vi "Generate Population.vi"(8 "error in (no error)":errorcluster, 9 "seed":i32=-1, 10 "OSSP_Problem.lvclass":refnum<class "OSSP_Problem.lvclass">, 11 "GA in":refnum<class "GA.lvclass">) -> (0 "error out":errorcluster, 3 "GA out":refnum<class "GA.lvclass">)   [LabVIEW 2013, in "GA.lvclass"]
uses:
  GA.lvclass
  OSSP_Problem.lvclass
  GA.lvclass/GA.ctl
  Controls/Solution_GA.ctl
  OSSP_Problem.lvclass/OSSP_Problem.ctl
  Helper VIs/IRH Heuristic VIs/Initial Construction Heuristic.ctl
  GA/Controls/Scheduler Type.ctl
  Scheduler_Class/Prins FIFO Scheduler Methods and Controls/Prins FIFO Scheduler.vi
  Scheduler_Class/Prins FIFO Scheduler Methods and Controls/Methods/Calculate Final Completion Times of Jobs.vi
  Scheduler_Class/Prins FIFO Scheduler Methods and Controls/Methods/Reorder Schedule(Prins FIFO) based on Start Times.vi
  OSSP_Problem_Class/Getters/Read Number of Jobs.vi
  OSSP_Problem_Class/Getters/Read Number of Machines.vi
  Scheduler_Class/NonDelay Scheduler/Non Delay Scheduler Engine.vi
  OSSP_Problem_Class/Getters/Read Due Dates.vi
  Scheduler_Class/Operation to Machine Job Tuple.vi
  <vilib>/dlg_ctls.llb/Space Constant.vi
  GA/SubVIS/Calcualte General Tardiness.vi
  Helper VIs/IRH Heuristic VIs/LPTSequenceBulilder.vi
  Helper VIs/IRH Heuristic VIs/SPTSequenceBulilder.vi
  Helper VIs/IRH Heuristic VIs/EDDSequenceBulilder.vi
  Scheduler_Class/Prins FIFO Scheduler Methods and Controls/Methods/UpdateMachineGaps.vi
  Scheduler_Class/Prins FIFO Scheduler Methods and Controls/Methods/UpdateJobGaps.vi
  Scheduler_Class/Prins FIFO Scheduler Methods and Controls/Methods/Find Intersecting Gaps.vi
  <vilib>/Analysis/1siggen.llb/Riffle Array (I32).vi
  Scheduler_Class/Prins FIFO Scheduler Methods and Controls/Methods/Transform to Plain Job and Machine Gaps Array.vi
  <vilib>/Analysis/NI_AALBase.lvlib
  Scheduler.lvclass
panel:
  out "Total Tardiness EDD":u16
  out "Total Tardiness SPT":u16
  out "Total Tardiness LPT":u16
  out "Schedule Out":i32[](array[numeric])
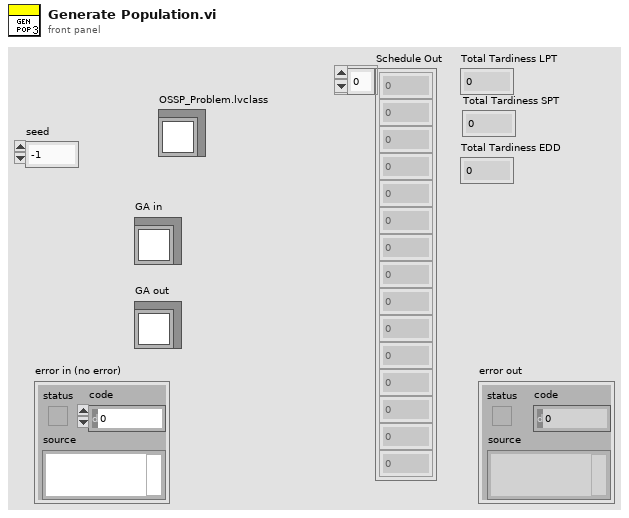
[diagram p1: front panel]
types:
  T1 = typedef "Solution_GA.ctl" = cluster{"Schedule":u16[], "Fitness":u16, "Fitness Valid?":bool}
  T2 = enum16{"Semi Active Scheduler", "Non Delay Scheduler"}
  T3 = typedef "Initial Construction Heuristic.ctl" = enum16{"LPT", "SPT", "EDD"}
  T4 = typedef "Objective.ctl" = enum16{"Makespan", "Total Tardiness"}
  T5 = typedef "GA.lvclass/Initial Population Generation.ctl" = enum16{"Random", "Heuristic Solution"}
  T6 = typedef "Scheduler Type.ctl" = enum16{"Non Delay Scheduler", "GT Active Scheduler", "My Faulty Scheduler", "Prins FIFO Scheduler", "SemiActive Scheduler"}
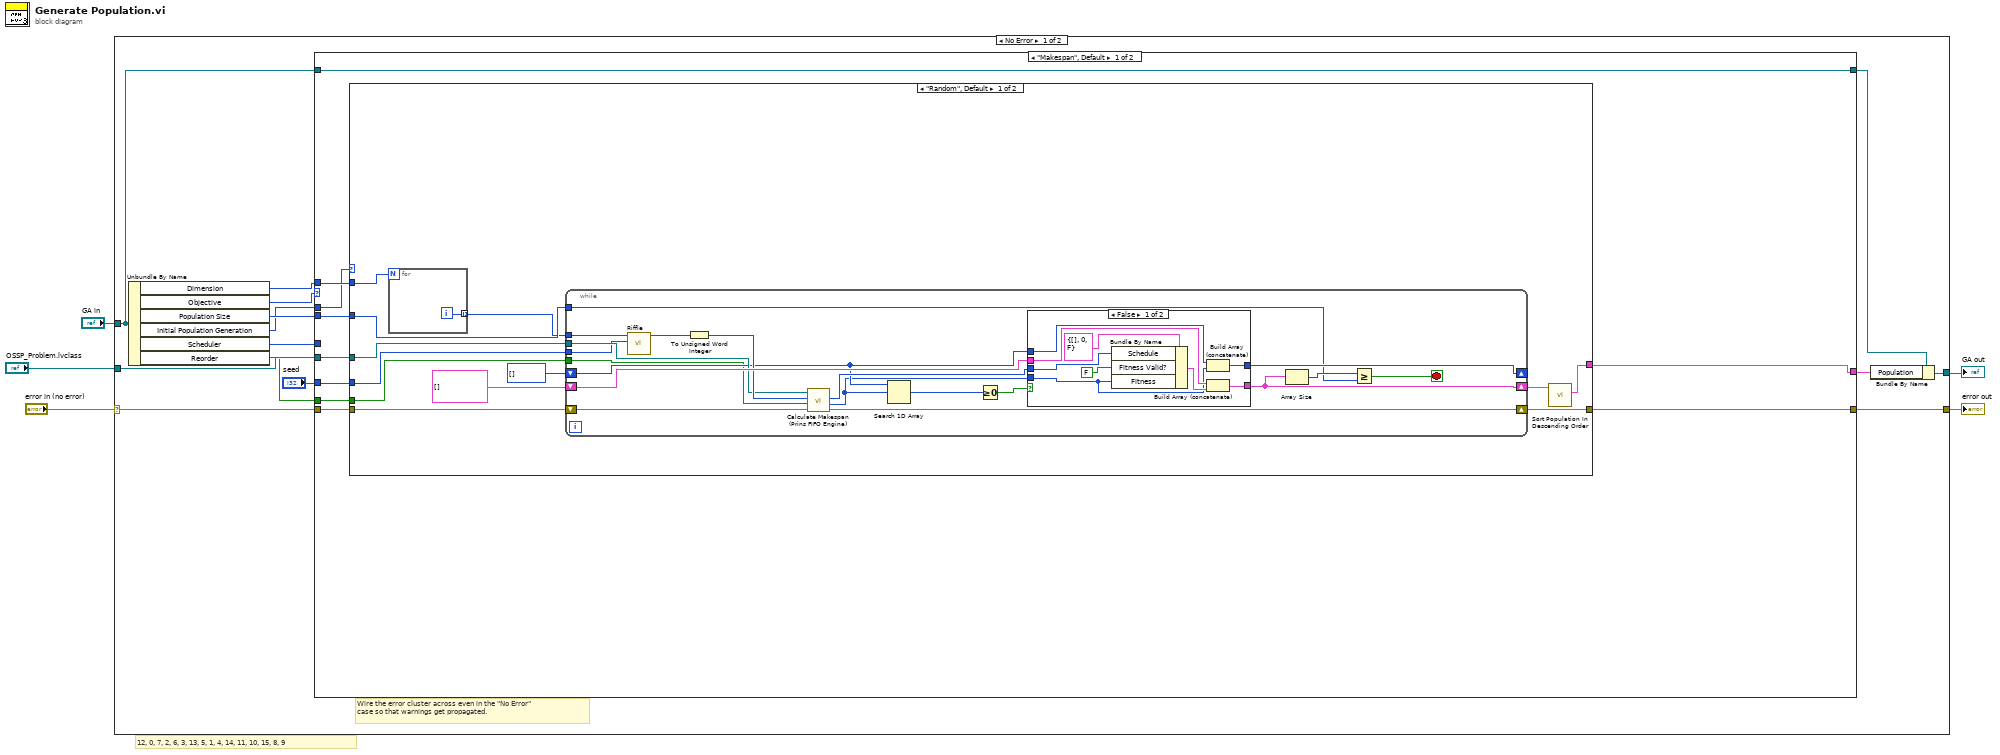
[diagram p0: block diagram]
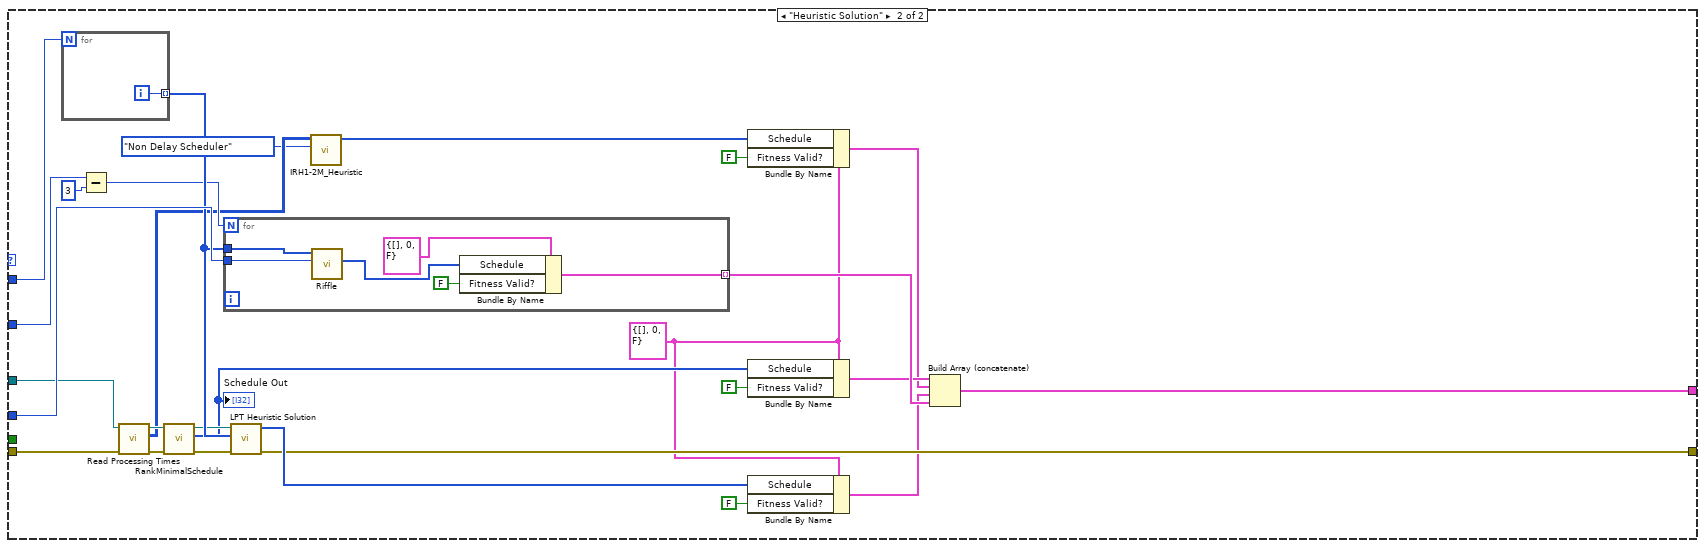
[diagram p3: hidden frame]
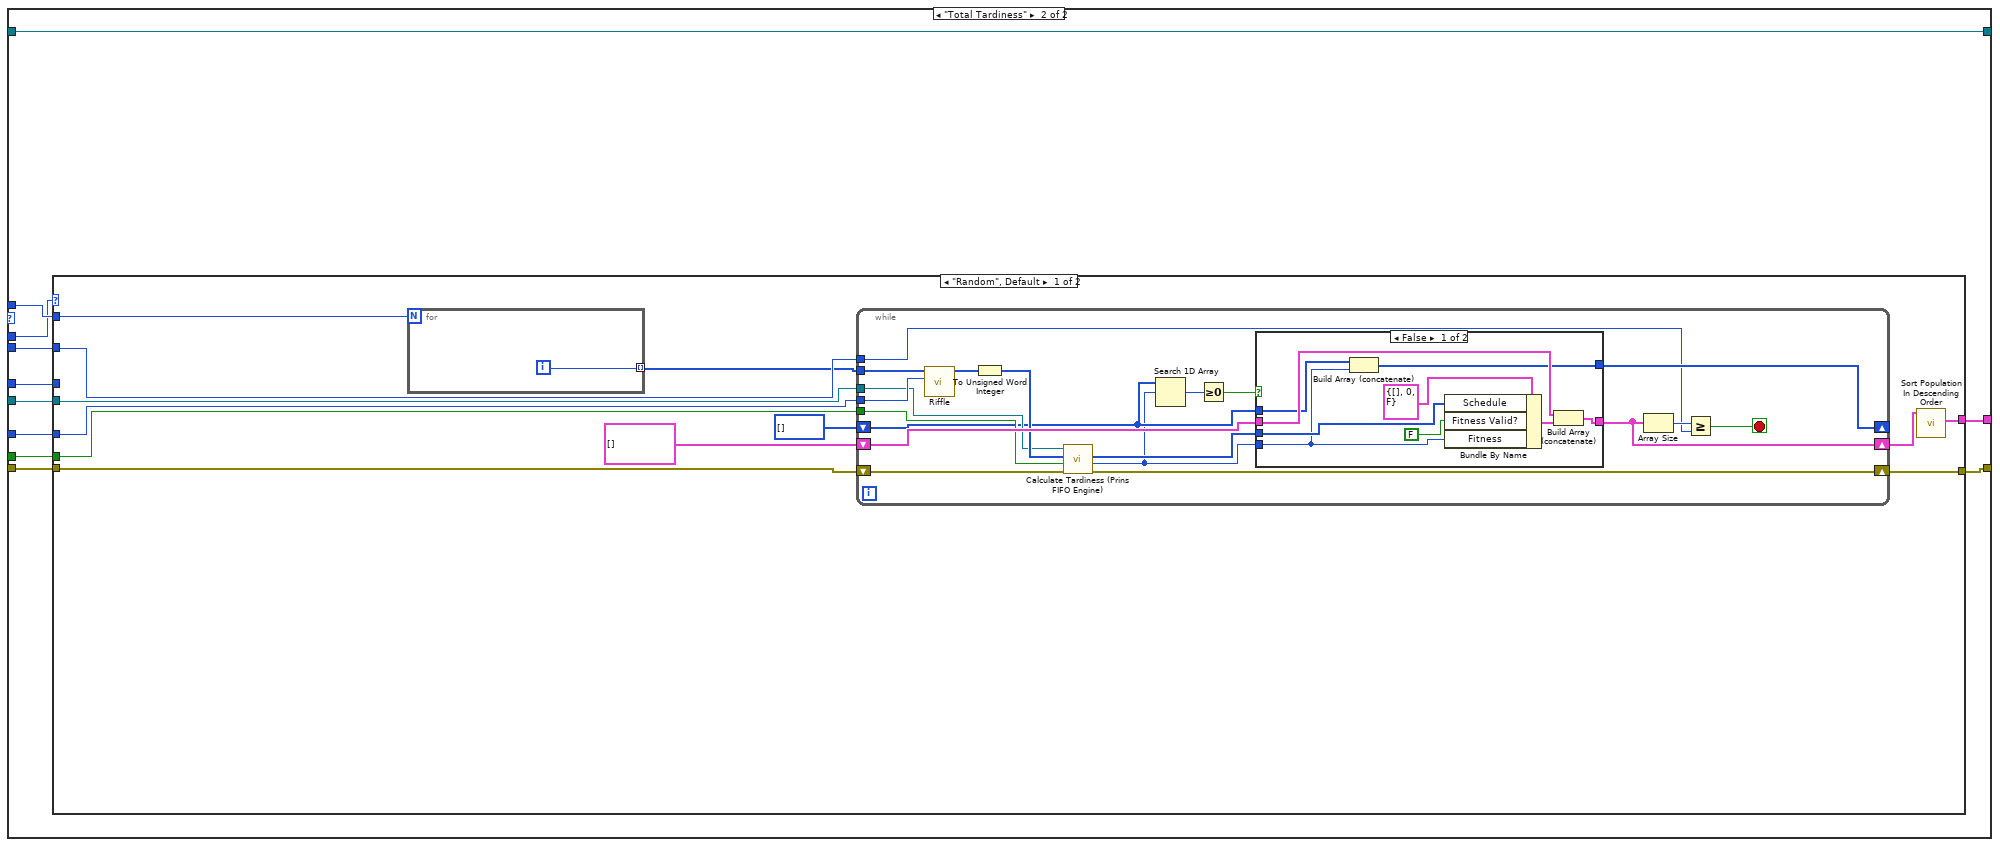
[diagram p4: hidden frame]
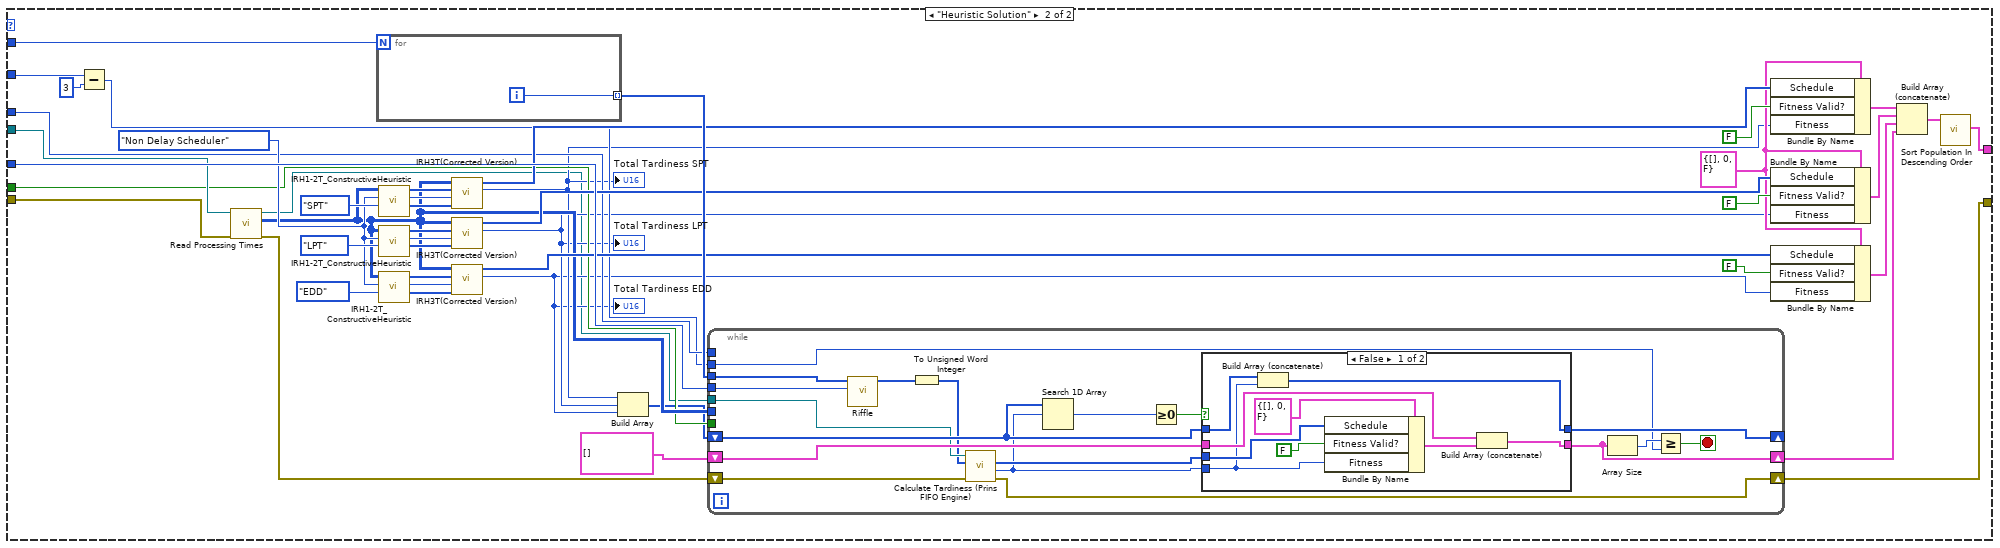
[diagram p6: hidden frame]
diagram:
  # "12, 0, 7, 2, 6, 3, 13, 5, 1, 4, 14, 11, 10, 15, 8, 9"
  n1 = case shown="No Error" "error in (no error)" {
    selector: "error in (no error)" -> [w12 w237]
    tunnel: [w14 w237] -> w4
    tunnel: [w18 w236] -> w2
    tunnel: "GA in" -> [w10 w236]
    tunnel: "OSSP_Problem.lvclass" -> [w11 _]
    frame No Error {
      # "Wire the error cluster across even in the \"No Error\"\ncase so that warnings get propagated."
      n2 = Unbundle By Name(w10) -> ("Dimension"=w19:i32, "Objective"=w15:T4, "Population Size"=w13:u32, "Initial Population Generation"=w8:T5, "Scheduler"=w7:T6, "Reorder"=w6:bool)
      n3 = case shown="\"Makespan\", Default" w15 {
        tunnel: w19 -> [w29 w117]
        tunnel: "seed" -> [w28 w116]
        tunnel: [w27 w114] -> w16
        tunnel: w11 -> [w24 w112]
        tunnel: w12 -> [w23 w115]
        tunnel: [w26 w111] -> w14
        tunnel: w13 -> [w25 w113]
        tunnel: w10 -> [w22 w110]
        tunnel: [w22 w110] -> w9
        tunnel: w8 -> [w21 w109]
        tunnel: w7 -> [_ w108]
        tunnel: w6 -> [w20 w107]
        frame "Makespan", Default {
          n4 = case shown="\"Random\", Default" w21 {
            tunnel: w29 -> [w33 w99]
            tunnel: w28 -> [w32 w98]
            tunnel: [w30 w95] -> w27
            tunnel: [w40 w92] -> w26
            tunnel: w25 -> [w38 w86]
            tunnel: w24 -> [w39 w83]
            tunnel: w23 -> [w41 w82]
            tunnel: w20 -> [w31 _]
            frame "Random", Default {
              n5 = for {
                N: w33 -> [_]
                tunnel: [w72] -> w37 mode=indexing
                i -> [w72]
              }
              n6 = while {
                tunnel: w37 -> [w60]
                tunnel: w38 -> [w50]
                shift-right: [w51] -> w34
                shift-left: T1[] [] -> [w53]
                shift-right: [w52] -> _
                shift-left: u16[] [] ("appended array") -> [w45]
                shift-right: [w48] -> w40
                shift-left: w41 -> [w49]
                tunnel: w39 -> [w46]
                tunnel: w32 -> [w43]
                tunnel: w31 -> [w42]
                stop <- w56 stop-if-true
                n7 = call-poly <vilib>:"Riffle.vi"("seed"=w43, "X"=w60) -> ("Riffled {X}"=w58:i32[])  [unwired: 7 in, 2 out]
                n8 = To Unsigned Word Integer(number=w58) -> (unsigned 16bit integer=w47:u16[])
                n9 = call "Calculate Makespan (Prins FIFO Engine).vi"("error in (no error)"=w49, "Reorder?"=w42, "Schedule In"=w47, "OSSP_Problem in"=w46) -> ("error out"=w48:errorcluster, "Makespan"=w44:i32, "Schedule Out"=w59:u16[])  [unwired: 4 in, 1 out]
                n10 = Search 1D Array(1D array=w45, element=w44) -> (index of element=w55:i32)  [unwired: 1 in]
                n11 = Greater Or Equal To 0?(x=w55) -> (x >= 0?=w54:bool)
                n12 = case shown="False" w54 {
                  tunnel: w59 -> [w67 _]
                  tunnel: w53 -> [w66 w71]
                  tunnel: [w64 w71] -> w51
                  tunnel: w45 -> [w63 w70]
                  tunnel: [w62 w70] -> w52
                  tunnel: w44 -> [w61 _]
                  frame False {
                    n13 = Bundle By Name(cluster=T1 {"Schedule"=[], "Fitness"=0, "Fitness Valid?"=FALSE} ("Solution"), "Schedule"=w67, "Fitness Valid?"=FALSE, "Fitness"=w61) -> (w65:T1)
                    n14 = Build Array (concatenate)(w63, w61) -> (w62:i32[])
                    n15 = Build Array (concatenate)(w66, w65) -> (w64:T1[])
                  }
                  frame True {
                  }
                }
                n16 = Array Size(array=w51) -> (size(s)=w57:i32)
                n17 = Greater Or Equal?(x=w57, y=w50) -> (x >= y?=w56:bool)
              }
              n18 = call "Sort Population In Descending Order.vi"("Population"=w34) -> ("Population In Descending Order"=w30:T1[])  [unwired: 9 in, 1 out]
            }
            frame "Heuristic Solution" {
              w77 = T1 {"Schedule"=[], "Fitness"=0, "Fitness Valid?"=FALSE} ("Solution")
              n19 = for {
                N: w99 -> [_]
                tunnel: [w100] -> w97 mode=indexing
                i -> [w100]
              }
              n20 = Subtract(x=w86, y=u8 3) -> (x-y=w84:u32)
              n21 = call "Read Processing Times.vi"("error in (no error)"=w82, "OSSP_Problem in"=w83) -> ("error out"=w81:errorcluster, "Processing Times"=w79:u16[][], "OSSP_Problem out"=w80:refnum<class "OSSP_Problem.lvclass">)  [unwired: 7 in]
              n22 = call "RankMinimalSchedule.vi"("error in (no error)"=w81, "OSSP_Problem in"=w80) -> ("error out"=w91:errorcluster, "Schedule Out"=w89:i32[], "OSSP_Problem out"=w90:refnum<class "OSSP_Problem.lvclass">)  [unwired: 7 in]
              "Schedule Out" <- w89
              n23 = for {
                N: w84 -> [_]
                tunnel: w97 -> [w106]
                tunnel: w98 -> [w105]
                tunnel: [w103] -> w96 mode=indexing
                n24 = call-poly <vilib>:"Riffle.vi"("seed"=w105, "X"=w106) -> ("Riffled Index"=w104:i32[])  [unwired: 7 in, 2 out]
                n25 = Bundle By Name(cluster=T1 {"Schedule"=[], "Fitness"=0, "Fitness Valid?"=FALSE} ("Solution"), "Schedule"=w104, "Fitness Valid?"=FALSE) -> (w103:T1)
              }
              n26 = call "LPT Heuristic Solution.vi"("error in (no error)"=w91, "Array"=w97, "OSSP_Problem in"=w90) -> ("error out"=w92:errorcluster, "LPT List Heuristic Solution"=w93:u16[])  [unwired: 7 in]
              n27 = call "IRH1-2M_Heuristic.vi"("Scheduler"=T2."Non Delay Scheduler", "Proocessing Times"=w79) -> ("IRH1 Schedule"=w73:u16[])  [unwired: 9 in]
              n28 = Bundle By Name(cluster=w77, "Schedule"=w73, "Fitness Valid?"=FALSE) -> (w75:T1)
              n29 = Bundle By Name(cluster=w77, "Schedule"=w89, "Fitness Valid?"=FALSE) -> (w87:T1)
              n30 = Bundle By Name(cluster=w77, "Schedule"=w93, "Fitness Valid?"=FALSE) -> (w74:T1)
              n31 = Build Array (concatenate)(w87, w75, w74, w96) -> (w95:T1[])
            }
          }
        }
        frame "Total Tardiness" {
          n32 = case shown="\"Random\", Default" w109 {
            tunnel: w117 -> [w129 w205]
            tunnel: w116 -> [w127 w204]
            tunnel: w115 -> [w124 w174]
            tunnel: [w122 w164] -> w114
            tunnel: w113 -> [w126 w203]
            tunnel: w112 -> [w125 w202]
            tunnel: [w123 w161] -> w111
            tunnel: w108 -> [_ w176]
            tunnel: w107 -> [w128 w173]
            frame "Random", Default {
              n33 = for {
                N: w129 -> [_]
                tunnel: [w160] -> w121 mode=indexing
                i -> [w160]
              }
              n34 = while {
                tunnel: w121 -> [w148]
                tunnel: w127 -> [w147]
                tunnel: w128 -> [w132]
                tunnel: w126 -> [w137]
                shift-right: [w138] -> w118
                shift-left: T1[] [] -> [w140]
                shift-right: [w139] -> _
                shift-left: u16[] [] ("appended array") -> [w131]
                shift-right: [w135] -> w123
                shift-left: w124 -> [w136]
                tunnel: w125 -> [w133]
                stop <- w143 stop-if-true
                n35 = call-poly <vilib>:"Riffle.vi"("seed"=w147, "X"=w148) -> ("Riffled {X}"=w145:i32[])  [unwired: 7 in, 2 out]
                n36 = To Unsigned Word Integer(number=w145) -> (unsigned 16bit integer=w134:u16[])
                n37 = call "Calculate Tardiness (Prins FIFO Engine).vi"("error in (no error)"=w136, "Reorder?"=w132, "Schedule In"=w134, "OSSP_Problem in"=w133) -> ("error out"=w135:errorcluster, "Tardiness(Prins FIFO Engine)"=w130:u16, "Schedule Out"=w146:u16[])  [unwired: 3 in, 2 out]
                n38 = Search 1D Array(1D array=w131, element=w130) -> (index of element=w142:i32)  [unwired: 1 in]
                n39 = Greater Or Equal To 0?(x=w142) -> (x >= 0?=w141:bool)
                n40 = case shown="False" w141 {
                  tunnel: w146 -> [w155 _]
                  tunnel: w140 -> [w154 w159]
                  tunnel: [w152 w159] -> w138
                  tunnel: w131 -> [w151 w158]
                  tunnel: [w150 w158] -> w139
                  tunnel: w130 -> [w149 _]
                  frame False {
                    n41 = Build Array (concatenate)(w151, w149) -> (w150:u16[])
                    n42 = Bundle By Name(cluster=T1 {"Schedule"=[], "Fitness"=0, "Fitness Valid?"=FALSE} ("Solution"), "Schedule"=w155, "Fitness Valid?"=FALSE, "Fitness"=w149) -> (w153:T1)
                    n43 = Build Array (concatenate)(w154, w153) -> (w152:T1[])
                  }
                  frame True {
                  }
                }
                n44 = Array Size(array=w138) -> (size(s)=w144:i32)
                n45 = Greater Or Equal?(x=w144, y=w137) -> (x >= y?=w143:bool)
              }
              n46 = call "Sort Population In Descending Order.vi"("Population"=w118) -> ("Population In Descending Order"=w122:T1[])  [unwired: 9 in, 1 out]
            }
            frame "Heuristic Solution" {
              w178 = Scheduler_Type."Non Delay Scheduler" ("Scheduler")
              w177 = T1 {"Schedule"=[], "Fitness"=0, "Fitness Valid?"=FALSE} ("Solution")
              n47 = Subtract(x=w203, y=u8 3) -> (x-y=w172:u32)
              n48 = call "Read Processing Times.vi"("error in (no error)"=w174, "OSSP_Problem in"=w202) -> ("error out"=w162:errorcluster, "Processing Times"=w175:u16[][], "OSSP_Problem out"=w163:refnum<class "OSSP_Problem.lvclass">)  [unwired: 7 in]
              n49 = for {
                N: w205 -> [_]
                tunnel: [w235] -> w201 mode=indexing
                i -> [w235]
              }
              n50 = call "IRH1-2T_ConstructiveHeuristic.vi"("Initial Construction Heursitic"=Initial_Construction_Heuristic."SPT", "Scheduler"=w178, "Proocessing Times MxJ"=w175) -> ("Due Dates"=w191:u16[], "Total Tardiness"=w192:u16, "IRH2T Schedule Out"=w193:u16[])  [unwired: 6 in]
              n51 = call "IRH1-2T_ConstructiveHeuristic.vi"("Initial Construction Heursitic"=Initial_Construction_Heuristic."LPT", "Scheduler"=w178, "Proocessing Times MxJ"=w175) -> ("Due Dates"=w196:u16[], "Total Tardiness"=w197:u16, "IRH2T Schedule Out"=w198:u16[])  [unwired: 6 in]
              n52 = call "IRH1-2T_ConstructiveHeuristic.vi"("Initial Construction Heursitic"=Initial_Construction_Heuristic."EDD", "Scheduler"=w178, "Proocessing Times MxJ"=w175) -> ("Due Dates"=w187:u16[], "Total Tardiness"=w188:u16, "IRH2T Schedule Out"=w189:u16[])  [unwired: 6 in]
              n53 = call "IRH3T(Corrected Version).vi"("Due Dates"=w191, "Initial Tardiness"=w192, "Schedule 2B Improved"=w193, "Proocessing Times  (Machines x Jobs)"=w175) -> ("Total Tardiness"=w169:u16, "IRH3T (Reordered) Schedule Out"=w183:u16[])  [unwired: 5 in, 1 out]
              "Total Tardiness SPT" <- w169
              n54 = call "IRH3T(Corrected Version).vi"("Due Dates"=w196, "Initial Tardiness"=w197, "Schedule 2B Improved"=w198, "Proocessing Times  (Machines x Jobs)"=w175) -> ("Total Tardiness"=w168:u16, "IRH3T (Reordered) Schedule Out"=w184:u16[])  [unwired: 5 in, 1 out]
              "Total Tardiness LPT" <- w168
              n55 = call "IRH3T(Corrected Version).vi"("Due Dates"=w187, "Initial Tardiness"=w188, "Schedule 2B Improved"=w189, "Proocessing Times  (Machines x Jobs)"=w175) -> ("Total Tardiness"=w167:u16, "IRH3T (Reordered) Schedule Out"=w182:u16[])  [unwired: 5 in, 1 out]
              "Total Tardiness EDD" <- w167
              n56 = Build Array(w169, w168, w167) -> (w166:u16[])
              n57 = while {
                tunnel: w201 -> [w223]
                tunnel: w204 -> [w222]
                tunnel: w176 -> [_]
                tunnel: w175 -> [_]
                tunnel: w163 -> [w210]
                tunnel: w173 -> [_]
                tunnel: w172 -> [w211]
                shift-right: [w212] -> w170
                shift-left: T1[] [] -> [w215]
                shift-right: [w213] -> _
                shift-left: w166 -> [w214]
                shift-right: [w208] -> w161
                shift-left: w162 -> [w209]
                stop <- w218 stop-if-true
                n58 = call-poly <vilib>:"Riffle.vi"("seed"=w222, "X"=w223) -> ("Riffled {X}"=w220:i32[])  [unwired: 7 in, 2 out]
                n59 = To Unsigned Word Integer(number=w220) -> (unsigned 16bit integer=w207:u16[])
                n60 = call "Calculate Tardiness (Prins FIFO Engine).vi"("error in (no error)"=w209, "Schedule In"=w207, "OSSP_Problem in"=w210) -> ("error out"=w208:errorcluster, "Tardiness(Prins FIFO Engine)"=w206:u16, "Schedule Out"=w221:u16[])  [unwired: 4 in, 2 out]
                n61 = Search 1D Array(1D array=w214, element=w206) -> (index of element=w217:i32)  [unwired: 1 in]
                n62 = Greater Or Equal To 0?(x=w217) -> (x >= 0?=w216:bool)
                n63 = case shown="False" w216 {
                  tunnel: w221 -> [w230 _]
                  tunnel: w215 -> [w229 w234]
                  tunnel: [w227 w234] -> w212
                  tunnel: w214 -> [w226 w233]
                  tunnel: [w225 w233] -> w213
                  tunnel: w206 -> [w224 _]
                  frame False {
                    n64 = Build Array (concatenate)(w226, w224) -> (w225:u16[])
                    n65 = Bundle By Name(cluster=T1 {"Schedule"=[], "Fitness"=0, "Fitness Valid?"=FALSE} ("Solution"), "Schedule"=w230, "Fitness Valid?"=FALSE, "Fitness"=w224) -> (w228:T1)
                    n66 = Build Array (concatenate)(w229, w228) -> (w227:T1[])
                  }
                  frame True {
                  }
                }
                n67 = Array Size(array=w212) -> (size(s)=w219:i32)
                n68 = Greater Or Equal?(x=w219, y=w211) -> (x >= y?=w218:bool)
              }
              n69 = Bundle By Name(cluster=w177, "Schedule"=w183, "Fitness Valid?"=FALSE, "Fitness"=w169) -> (w180:T1)
              n70 = Bundle By Name(cluster=w177, "Schedule"=w184, "Fitness Valid?"=FALSE, "Fitness"=w168) -> (w179:T1)
              n71 = Bundle By Name(cluster=w177, "Schedule"=w182, "Fitness Valid?"=FALSE, "Fitness"=w167) -> (w181:T1)
              n72 = Build Array (concatenate)(w180, w179, w181, w170) -> (w165:T1[])
              n73 = call "Sort Population In Descending Order.vi"("Population"=w165) -> ("Population In Descending Order"=w164:T1[])  [unwired: 9 in, 1 out]
            }
          }
        }
      }
      n74 = Bundle By Name(cluster=w9, "Population"=w16) -> (w18:refnum<class "GA.lvclass">)
    }
    frame Error {
    }
  }
  "error out" <- w4
  "GA out" <- w2
